vi "TL init IR sensors.vi"() -> (0 "IR Sensors":T1(array[cluster]))   [LabVIEW 2014]
doc: "This vi initiates the IR sensors as an array of clusters with Name, local angle direction, and distance reading. A reading of 0.0 is meant to be no object found."
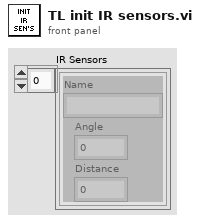
[diagram p1: front panel]
types:
  T1 = cluster{"Name":string, "Angle":dbl, "Distance":dbl}[]
  T2 = cluster{"Name":string, "Angle":dbl, "Distance":dbl}
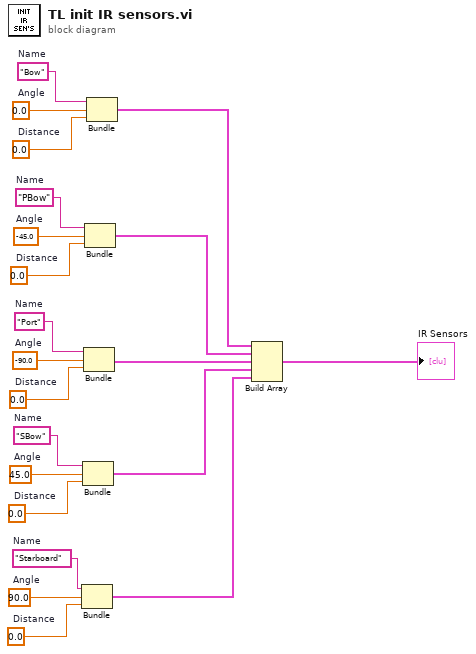
[diagram p0: block diagram]
diagram:
  w7 = 0.0  # Distance
  w9 = 90.0  # Angle
  w8 = "Starboard"  # Name
  w10 = 0.0  # Distance
  w12 = 45.0  # Angle
  w11 = "SBow"  # Name
  w13 = 0.0  # Distance
  w15 = -90.0  # Angle
  w14 = "Port"  # Name
  w16 = 0.0  # Distance
  w18 = -45.0  # Angle
  w17 = "PBow"  # Name
  w19 = 0.0  # Distance
  w21 = 0.0  # Angle
  w20 = "Bow"  # Name
  n1 = Bundle("Name"=w8, "Angle"=w9, "Distance"=w7) -> (w2:T2)  [unwired: 1 in]
  n2 = Bundle("Name"=w11, "Angle"=w12, "Distance"=w10) -> (w3:T2)  [unwired: 1 in]
  n3 = Bundle("Name"=w14, "Angle"=w15, "Distance"=w13) -> (w4:T2)  [unwired: 1 in]
  n4 = Bundle("Name"=w17, "Angle"=w18, "Distance"=w16) -> (w5:T2)  [unwired: 1 in]
  n5 = Bundle("Name"=w20, "Angle"=w21, "Distance"=w19) -> (w6:T2)  [unwired: 1 in]
  n6 = Build Array(w6, w5, w4, w3, w2) -> (→"IR Sensors":T1)
